vi "zadanie6_2.vi"() -> ()   [LabVIEW 2012]
panel:
  out "Tablica wyników cała 2":dbl[][][][][](array[numeric]) caption="Array 2"
  out "Tablica wyników cała":dbl[][][][][](array[numeric]) caption="Array 2"
  out "Tablica wyników":dbl[][](array[numeric])
  # "Program oblicza wartości y(x) = 1 - e^(-x) dla x = {0.1 , 0.2, 0.3, .... , 4.8, 4.9, 5.0}"
  # "x"
  # "y"
  # "x"
  # "y"
  # "x"
  # "y"
  # "x"
  # "y"
  # "x"
  # "y"
  # "x"
  # "y"
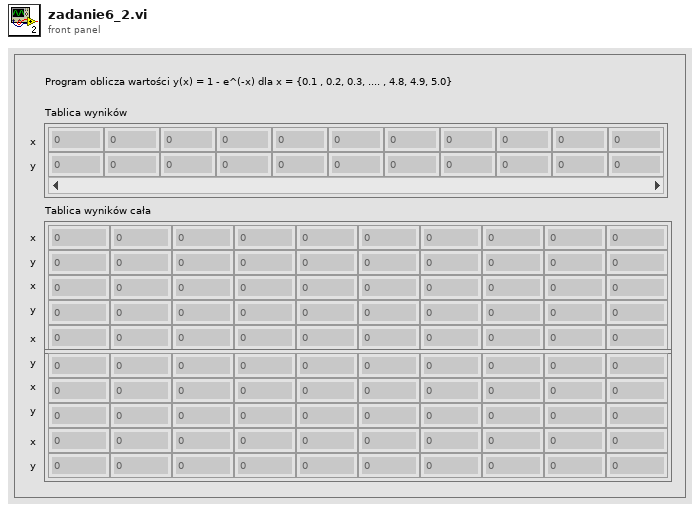
[diagram p1: front panel]
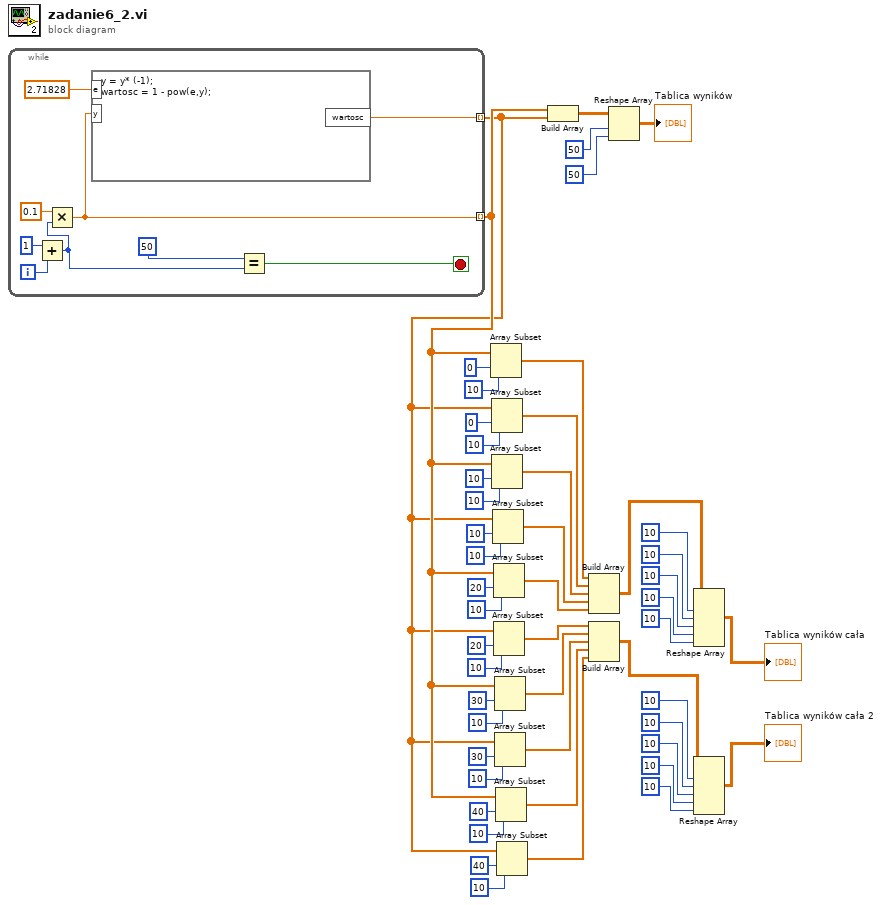
[diagram p0: block diagram]
diagram:
  n1 = while {
    tunnel: [w58] -> w20 mode=indexing
    tunnel: [w57] -> w19 mode=indexing
    i -> [w52]
    stop <- w55 stop-if-true
    n2 = Add(x=1, y=w52) -> (x+y=w51:i32)
    n3 = Multiply(x=0.1, y=w51) -> (x*y=w58:dbl)
    n4 = formula code="y = y* (-1);\nwartosc = 1 - pow(e,y);"("y"=w58, "e"=2.71828) -> ("wartosc"=w57:dbl)
    n5 = Equal?(x=50, y=w51) -> (x = y?=w55:bool)
  }
  n6 = Array Subset(array=w20, index=0, length=10) -> (w18:dbl[])
  n7 = Array Subset(array=w19, index=0, length=10) -> (w17:dbl[])
  n8 = Array Subset(array=w20, index=10, length=10) -> (w16:dbl[])
  n9 = Array Subset(array=w19, index=10, length=10) -> (w15:dbl[])
  n10 = Array Subset(array=w20, index=20, length=10) -> (w14:dbl[])
  n11 = Array Subset(array=w19, index=20, length=10) -> (w8:dbl[])
  n12 = Array Subset(array=w20, index=30, length=10) -> (w7:dbl[])
  n13 = Array Subset(array=w19, index=30, length=10) -> (w6:dbl[])
  n14 = Array Subset(array=w20, index=40, length=10) -> (w5:dbl[])
  n15 = Array Subset(array=w19, index=40, length=10) -> (w4:dbl[])
  n16 = Build Array(w20, w19) -> (w50:dbl[][])
  n17 = Build Array(w18, w17, w16, w15, w14) -> (w46:dbl[][])
  n18 = Build Array(w8, w7, w6, w5, w4) -> (w3:dbl[][])
  n19 = Reshape Array(w50, 50, 50) -> (→"Tablica wyników":dbl[][])
  n20 = Reshape Array(w46, 10, 10, 10, 10, 10) -> (→"Tablica wyników cała":dbl[][][][][])
  n21 = Reshape Array(w3, 10, 10, 10, 10, 10) -> (→"Tablica wyników cała 2":dbl[][][][][])
